vi "maillist.vi"() -> ()   [LabVIEW 2022 SP3]
panel:
  out "text":string
  out "String":string
  in  "file (use dialog)":path
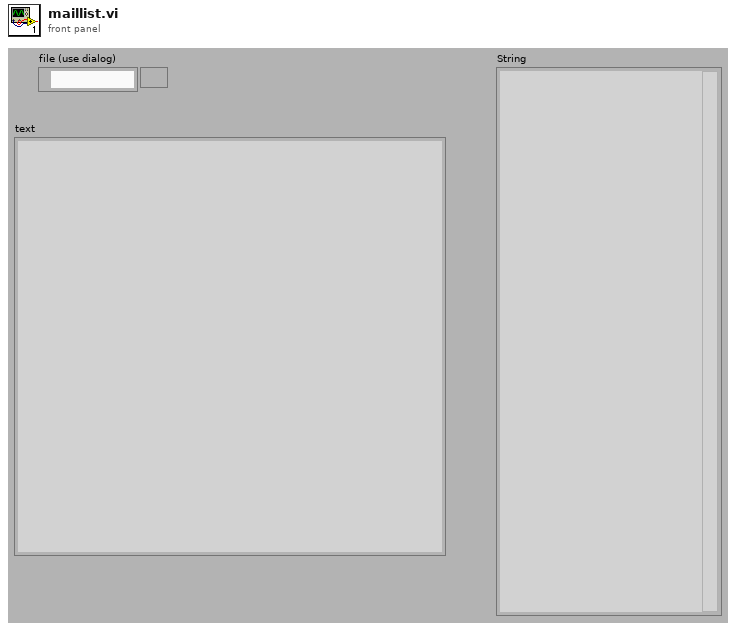
[diagram p1: front panel]
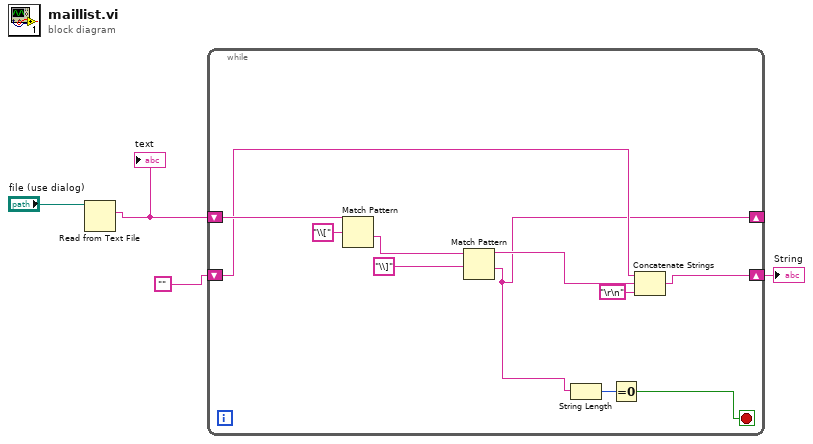
[diagram p0: block diagram]
diagram:
  n1 = Read from Text File(file (use dialog)="file (use dialog)") -> (text=w3:string)  [unwired: 3 in, 3 out]
  "text" <- w3
  n2 = while {
    shift-right: [w5] -> _
    shift-left: w3 -> [w15]
    shift-right: [w6] -> w1
    shift-left: "" -> [w8]
    stop <- w10 stop-if-true
    n3 = Match Pattern(string=w15, regular expression="\\[") -> (after substring=w13:string)  [unwired: 1 in, 3 out]
    n4 = Match Pattern(string=w13, regular expression="\\]") -> (before substring=w7:string, after substring=w5:string)  [unwired: 1 in, 2 out]
    n5 = String Length(string=w5) -> (length=w11:i32)
    n6 = Equal To 0?(x=w11) -> (x = 0?=w10:bool)
    n7 = Concatenate Strings(w8, w7, "\r\n") -> (w6:string)
  }
  "String" <- w1
